vi "Load Configuration From File.vi"(8 "error in (no error)":errorcluster, 9 "Name (Instance)":string, 10 "Configuration Path":path, 11 "System Actor in":refnum<class "System Actor.lvclass">) -> (0 "error out":errorcluster, 2 "Unflattened":string, 3 "System Actor out":refnum<class "System Actor.lvclass">)   [LabVIEW 2014, in "Robot Actor Framework.lvlib" / "System Actor.lvlib" / "System Actor.lvclass"]
uses:
  System Actor.lvclass
  System Actor.lvclass/System Actor.ctl
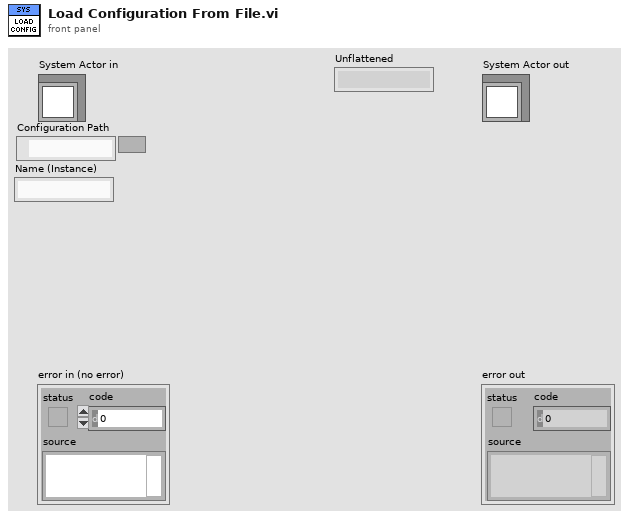
[diagram p1: front panel]
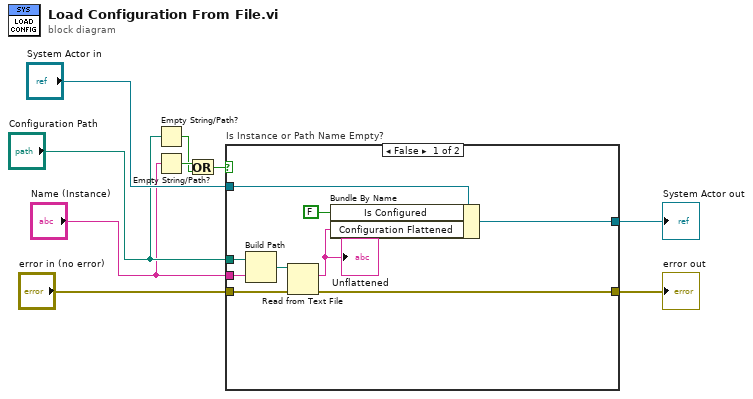
[diagram p0: block diagram]
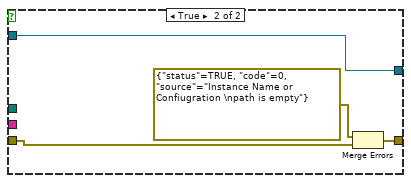
[diagram p2: hidden frame]
diagram:
  n1 = Empty String/Path?(string/path="Configuration Path") -> (empty?=w2:bool)
  n2 = Empty String/Path?(string/path="Name (Instance)") -> (empty?=w3:bool)
  n3 = Or(x=w3, y=w2) -> (x .or. y?=w1:bool)
  n4 = case "Is Instance or Path Name Empty?" shown="False" w1 {
    tunnel: "System Actor in" -> [w18 w19]
    tunnel: "Configuration Path" -> [w17 _]
    tunnel: "Name (Instance)" -> [w14 _]
    tunnel: [w13 w19] -> w6
    tunnel: "error in (no error)" -> [w12 w22]
    tunnel: [w11 w21] -> w8
    frame False {
      n5 = Build Path(base path=w17, name or relative path=w14) -> (appended path=w16:path)
      n6 = Read from Text File(file (use dialog)=w16, error in=w12) -> (text=w10:string, error out=w11:errorcluster)  [unwired: 2 in, 2 out]
      "Unflattened" <- w10
      n7 = Bundle By Name(cluster=w18, "Is Configured"=FALSE, "Configuration Flattened"=w10) -> (w13:refnum<class "System Actor.lvclass">)
    }
    frame True {
      n8 = Merge Errors(errorcluster {"status"=TRUE, "code"=0, "source"="Instance Name or Confiugration \npath is empty"} ("error in"), w22) -> (w21:errorcluster)
    }
  }
  "error out" <- w8
  "System Actor out" <- w6
